vi "tm3samp_sequence_triggermode.vi"() -> ()   [LabVIEW 2011]
panel:
  in  "Output Trigger":T1={"Mode"=1, "Polarity"=1, "Period"=0.0, "Delay"=0.0} {"Polarity" items=["Negative"=1, "Positive"=2]; "Mode" items=["Low"=1, "Global Exposure"=2, "Programmable"=3, "Trigger Ready"=4, "High"=5]}
  in  "Input Trigger":T2={"Mode"=1, "Polarity"=1, "Times"=1, "Delay"=0.0} {"Polarity" items=["Negative"=1, "Positive"=2]; "Mode" items=["Internal"=1, "External Edge"=2, "External Level"=4, "Software"=32, "Fast Repetition"=64, "TDI"=128, "Trigger Start"=512, "Sync Readout"=1024]}
  out "Image":u16[][](graph)
  out "Frames Per Second":dbl
  in  "Quit":bool
  out "Error Out":errorcluster
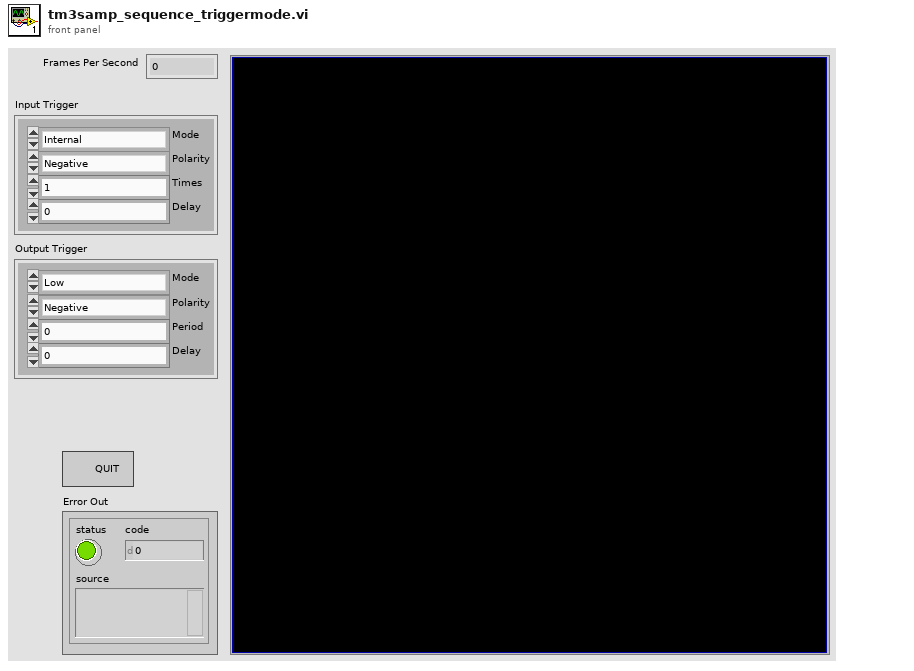
[diagram p1: front panel]
types:
  T1 = cluster{"Mode":u32, "Polarity":u32, "Period":dbl, "Delay":dbl}
  T2 = cluster{"Mode":u32, "Polarity":u32, "Times":u32, "Delay":dbl}
  T3 = cluster{"width":u32, "height":u32, "datatype":u32}
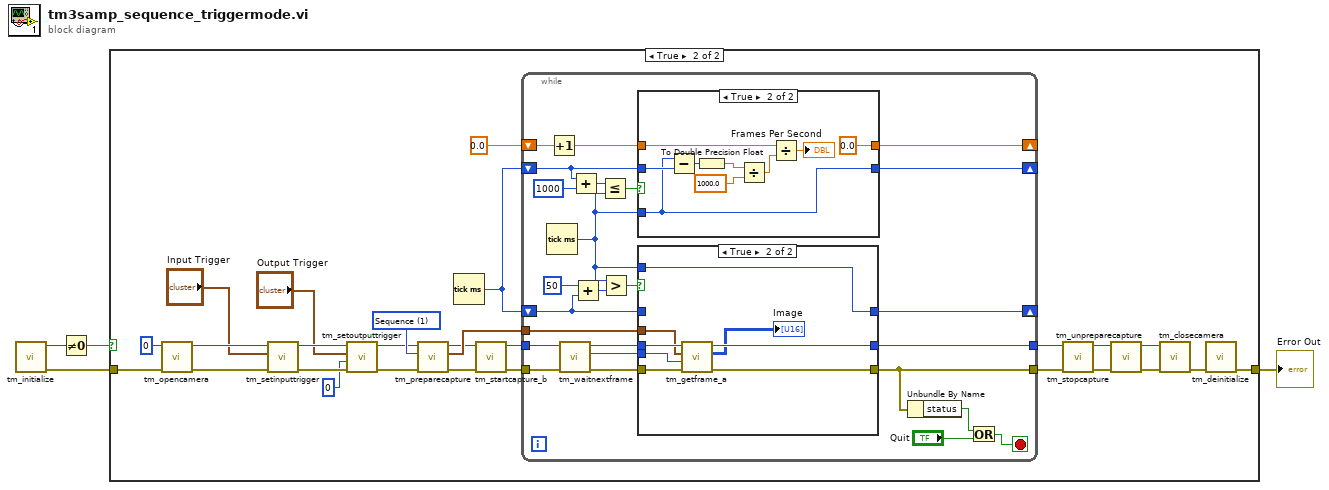
[diagram p0: block diagram]
diagram:
  n1 = call <userlib>:"tm_initialize.vi"() -> ("error out"=w1:errorcluster, "Number Of Cameras"=w2:u32)  [unwired: 10 in]
  n2 = Not Equal To 0?(x=w2) -> (x != 0?=w4:bool)
  n3 = case shown="True" w4 {
    tunnel: w1 -> [w5 w32]
    tunnel: [w5 w29] -> w3
    frame False {
    }
    frame True {
      w20 = 1 items=["Snap", "Sequence"] ("Capture mode")
      n4 = call <userlib>:"tm_opencamera.vi"("error in (no error)"=w32, "Camera Index"=u32 0) -> ("error out"=w10:errorcluster, "Handle out"=w11:u32)  [unwired: 8 in]
      n5 = call <userlib>:"tm_setinputtrigger.vi"("error in (no error)"=w10, "Parameters"="Input Trigger", "Handle in"=w11) -> ("error out"=w13:errorcluster, "Handle out"=w14:u32)  [unwired: 7 in]
      n6 = call <userlib>:"tm_setoutputtrigger.vi"("error in (no error)"=w13, "Index"=0, "Parameters"="Output Trigger", "Handle in"=w14) -> ("error out"=w8:errorcluster, "Handle out"=w9:u32)  [unwired: 6 in]
      n7 = call <userlib>:"tm_preparecapture.vi"("error in (no error)"=w8, "Capture mode"=w20, "Handle in"=w9) -> ("error out"=w17:errorcluster, "Buffer"=w19:T3, "Handle out"=w18:u32)  [unwired: 5 in, 1 out]
      n8 = Tick Count (ms)() -> (millisecond timer value=w15:u32)
      n9 = call <userlib>:"tm_startcapture_b.vi"("error in (no error)"=w17, "Handle in"=w18) -> ("error out"=w21:errorcluster, "Handle out"=w22:u32)  [unwired: 8 in]
      n10 = while {
        tunnel: [w36] -> w25
        tunnel: [w37] -> w26
        tunnel: w19 -> [w34]
        tunnel: w22 -> [w54]
        tunnel: w21 -> [w55]
        shift-right: [w52] -> _
        shift-left: w15 -> [w49]
        shift-right: [w53] -> _
        shift-left: 0.0 -> [w46]
        shift-right: [w35] -> _
        shift-left: w15 -> [w38]
        stop <- w33 stop-if-true
        n11 = Tick Count (ms)() -> (millisecond timer value=w39:u32)
        n12 = Increment(x=w46) -> (x+1=w47:dbl)
        n13 = call <userlib>:"tm_waitnextframe.vi"("error in (no error)"=w55, "Handle in"=w54) -> ("error out"=w44:errorcluster, "Frame Index"=w43:i32, "Handle out"=w45:u32)  [unwired: 6 in, 1 out]
        n14 = Add(x=w49, y=u32 1000) -> (x+y=w51:u32)
        n15 = Add(x=u32 50, y=w38) -> (x+y=w41:u32)
        n16 = Less Or Equal?(x=w51, y=w39) -> (x <= y?=w48:bool)
        n17 = Greater?(x=w39, y=w41) -> (0:w40:bool)
        n18 = case shown="True" w48 {
          tunnel: w49 -> [w70 w73]
          tunnel: [w70 w71] -> w52
          tunnel: w47 -> [w69 w77]
          tunnel: w39 -> [_ w71]
          tunnel: [w69 0.0] -> w53
          frame False {
          }
          frame True {
            n19 = Subtract(x=w71, y=w73) -> (x-y=w72:u32)
            n20 = To Double Precision Float(number=w72) -> (double precision float=w79:dbl)
            n21 = Divide(x=w79, y=1000.0) -> (x/y=w76:dbl)
            n22 = Divide(x=w77, y=w76) -> (x/y=→"Frames Per Second":dbl)
          }
        }
        n23 = case shown="True" w40 {
          tunnel: w45 -> [w60 w68]
          tunnel: w44 -> [w59 w67]
          tunnel: w43 -> [_ w66]
          tunnel: w38 -> [w58 _]
          tunnel: w39 -> [_ w65]
          tunnel: [w60 w62] -> w36
          tunnel: [w59 w63] -> w37
          tunnel: [w58 w65] -> w35
          tunnel: w34 -> [_ w64]
          frame False {
          }
          frame True {
            n24 = call <userlib>:"tm_getframe_a.vi"("error in (no error)"=w67, "Frame Index"=w66, "Buffer"=w64, "Handle in"=w68) -> ("error out"=w63:errorcluster, "Data 16"=→"Image":u16[][], "Handle out"=w62:u32)  [unwired: 3 in, 2 out]
          }
        }
        n25 = Unbundle By Name(w37) -> ("status"=w57:bool)
        n26 = Or(x=w57, y="Quit") -> (x .or. y?=w33:bool)
      }
      n27 = call <userlib>:"tm_stopcapture.vi"("error in (no error)"=w26, "Handle in"=w25) -> ("error out"=w23:errorcluster, "Handle out"=w24:u32)  [unwired: 8 in]
      n28 = call <userlib>:"tm_unpreparecapture.vi"("error in (no error)"=w23, "Handle in"=w24) -> ("error out"=w28:errorcluster, "Handle out"=w27:u32)  [unwired: 8 in]
      n29 = call <userlib>:"tm_closecamera.vi"("error in (no error)"=w28, "Handle in"=w27) -> ("error out"=w30:errorcluster)  [unwired: 9 in]
      n30 = call <userlib>:"tm_deinitialize.vi"("error in (no error)"=w30) -> ("error out"=w29:errorcluster)  [unwired: 10 in]
    }
  }
  "Error Out" <- w3
